vi "ADI_IMU_ADIS16448_RefNum Registry Get.vi"(8 "error in (no error)":errorcluster, 11 "refnum name":string="ADIIMURefNum") -> (0 "error out":errorcluster, 3 "ADI IMU DevRef":T1={"DevStatus"={"status"=FALSE, "code"=0, "source"=""}, "Handle"=0, "SPI Bus"=enum."SPI On-Board, CS0", "Device Found"=FALSE, "Device Ready"=FALSE, "Yaw Axis"=enum."Z", "AHRS Algorithm"=enum."Complementary", "Serial"=0, "Lot ID 2"=0, "Lot ID 1"=0, "Bytes Per Sample"=0, "Calibrate On Open?"=FALSE})   [LabVIEW 2018, in "ADIS16448_IMU.lvlib"]
doc: "Use this to get the reference you specify. You first must set the reference using RefNum Registry Set.vi."
uses:
  ADIS16448_IMU.lvlib
  ADI_IMU_ADIS16448_IMUDevRef.ctl
  <vilib>/Rock Robotics/SystemInterfaces/spilib/spi_bus.ctl
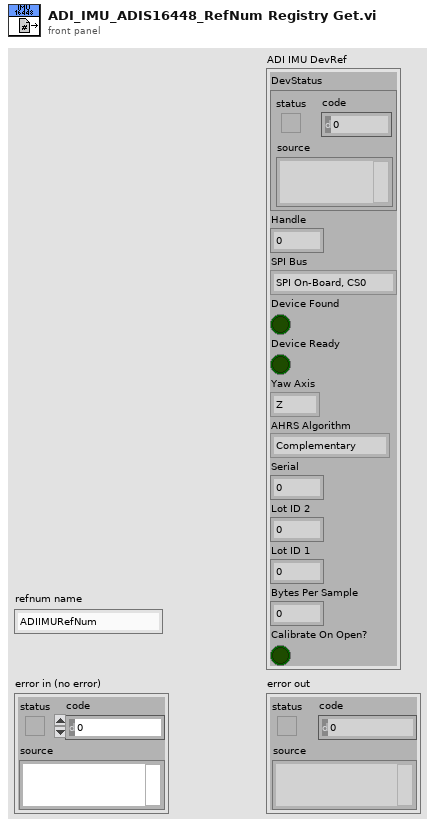
[diagram p1: front panel]
types:
  T1 = typedef "ADIS16448_IMU.lvlib/ADI_IMU_ADIS16448_IMUDevRef.ctl" = cluster{"DevStatus":errorcluster, "Handle":i32, "SPI Bus":T2, "Device Found":bool, "Device Ready":bool, "Yaw Axis":enum16{"X", "Y", "Z"}, "AHRS Algorithm":enum16{"Complementary", "Madgwick"}, "Serial":u16, "Lot ID 2":u16, "Lot ID 1":u16, "Bytes Per Sample":u16, "Calibrate On Open?":bool}
  T2 = typedef "spi_bus.ctl" = enum16{"SPI On-Board, CS0", "SPI On-Board, CS1", "SPI On-Board, CS2", "SPI On-Board, CS3", "SPI MXP", "Invalid"}
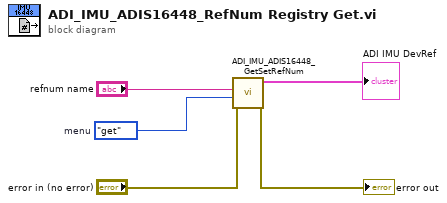
[diagram p0: block diagram]
diagram:
  w3 = enum16{"set", "get", "delete"}."get"  # menu
  n1 = call "ADI_IMU_ADIS16448_GetSetRefNum.vi"("error in (no error)"="error in (no error)", "menu"=w3, "refnum name"="refnum name") -> ("error out"=→"error out":errorcluster, "ADI IMU DevRef Get"=→"ADI IMU DevRef":T1)  [unwired: 7 in]
